vi "Material-Application-Dir-Support.vi"(0 "Support Resource Relative Filepath":string, 11 "error in":errorcluster) -> (4 "Support Filepath":path, 15 "error out":errorcluster)   [LabVIEW 2013]
panel:
  # "Inputs"
  # "Outputs"
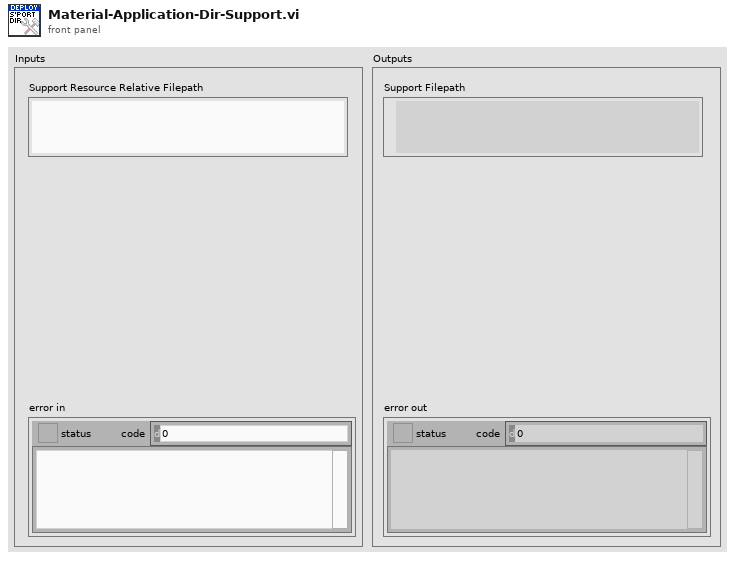
[diagram p1: front panel]
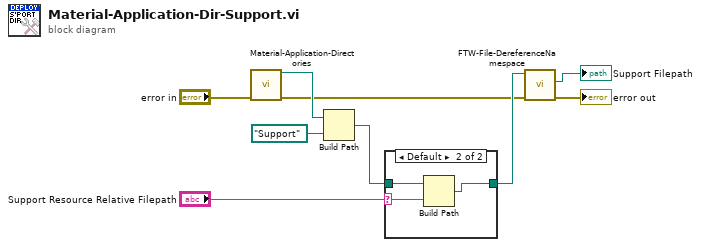
[diagram p0: block diagram]
diagram:
  n1 = call "Material-Application-Directories.vi"("error in"="error in") -> ("Deploy Root"=w7:path, "error out"=w2:errorcluster)  [unwired: 12 in, 1 out]
  n2 = Build Path(base path=w7, name or relative path=path "Support") -> (appended path=w6:path)
  n3 = case shown="Default" "Support Resource Relative Filepath" {
    selector: "Support Resource Relative Filepath" -> [_ w11]
    tunnel: [w10 w13] -> w4
    tunnel: w6 -> [w10 w12]
    frame "" {
    }
    frame Default {
      n4 = Build Path(base path=w12, name or relative path=w11) -> (appended path=w13:path)
    }
  }
  n5 = call "FTW-File-DereferenceNamespace.vi"("error in"=w2, "Base Filepath"=w4) -> ("error out"=→"error out":errorcluster, "Actual Filepath"=→"Support Filepath":path)  [unwired: 8 in]
